vi "coord_to_square.vi"(1 "Size":cluster{"x":dbl, "y":dbl}={"x"=40.0, "y"=40.0}, 3 "Centre":cluster{"x":dbl, "y":dbl}) -> (0 "rectangle":cluster{dbl, dbl, dbl, dbl})   [LabVIEW 2019]
doc: "This VI takes a point and a size (defaults to 40x40) and outputs l,t,r,b in a cluster to draw a rectangle (or extract an ROI)."
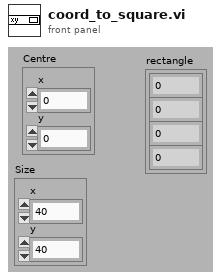
[diagram p1: front panel]
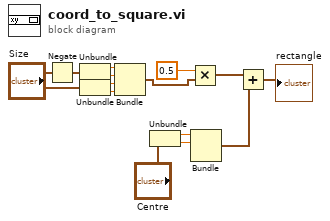
[diagram p0: block diagram]
diagram:
  n1 = Negate(x="Size") -> (-x=w4:cluster{"x":dbl, "y":dbl})
  n2 = Unbundle(w4) -> ("x"=w6:dbl, "y"=w5:dbl)
  n3 = Unbundle("Size") -> ("x"=w3:dbl, "y"=w2:dbl)
  n4 = Bundle("x"=w6, "y"=w5, "x"=w3, "y"=w2) -> (w7:cluster{"x":dbl, "y":dbl, "x":dbl, "y":dbl})  [unwired: 1 out]
  n5 = Unbundle("Centre") -> ("x"=w10:dbl, "y"=w11:dbl)
  n6 = Multiply(x=0.5, y=w7) -> (x*y=w9:cluster{"x":dbl, "y":dbl, "x":dbl, "y":dbl})
  n7 = Bundle("x"=w10, "y"=w11, "x"=w10, "y"=w11) -> (w12:cluster{"x":dbl, "y":dbl, "x":dbl, "y":dbl})  [unwired: 1 out]
  n8 = Add(x=w9, y=w12) -> (x+y=→"rectangle":cluster{"x":dbl, "y":dbl, "x":dbl, "y":dbl})
